vi "Get-Connection-Count.vi"() -> (3 "NumOfConnections":u32)   [LabVIEW 2017]
uses:
  Globals.vi
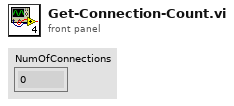
[diagram p1: front panel]
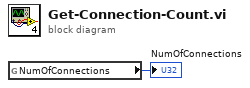
[diagram p0: block diagram]
diagram:
  n1 = global read "Globals.vi" "NumOfConnections"() -> (→"NumOfConnections":u32)
